vi "OpenListToINconList.vi"(11 "RVCLibrary_Bug2 in":refnum<class "RVCLibrary_Bug2.lvclass">) -> (3 "RVCLibrary_Bug2 out":refnum<class "RVCLibrary_Bug2.lvclass">)   [LabVIEW 2013, in "RVCLibrary_Bug2.lvclass"]
uses:
  RVCLibrary_Bug2.lvclass
  RVCLibrary_Bug2.lvclass/RVCLibrary_Bug2.ctl
  <vilib>/robotics/Navigation/shared/MapNode/AbstractDstarNode/NI_Robotics_AbstractDstarNode.lvclass
  <vilib>/robotics/Navigation/shared/Priority Queue/NI_Robotics_Priority Queue.lvclass
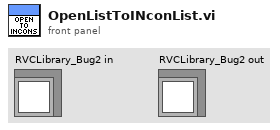
[diagram p1: front panel]
types:
  T1 = typedef "NI_Robotics_Priority Queue.lvclass/Open List Element.ctl" = cluster{"f":dbl, "g":dbl, "node Ref":refnum<data-value>}
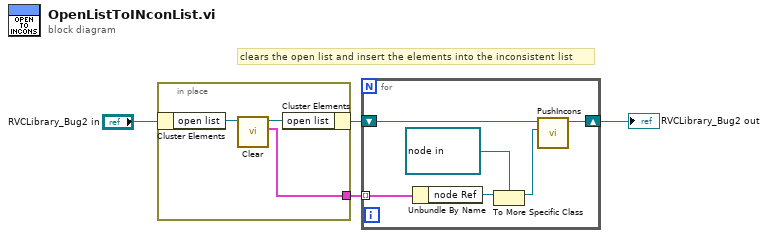
[diagram p0: block diagram]
diagram:
  # "clears the open list and insert the elements into the inconsistent list"
  n1 = in-place {
    in-place-border: [w5] -> w3
    n2 = in-place-cluster #1("RVCLibrary_Bug2 in") -> ("open list"=w7:refnum<class "NI_Robotics_Priority Queue.lvclass">)
    n3 = call <vilib>:"Clear.vi"("Priority Queue in"=w7) -> ("Open List"=w5:T1[], "Priority Queue out"=w6:refnum<class "NI_Robotics_Priority Queue.lvclass">)  [unwired: 8 in, 1 out]
    n4 = in-place-cluster #1("open list"=w6) -> (w4:refnum<class "RVCLibrary_Bug2.lvclass">)
  }
  n5 = for {
    tunnel: w3 -> [w12] mode=indexing
    shift-right: [w13] -> w2
    shift-left: w4 -> [w8]
    n6 = Unbundle By Name(w12) -> ("node Ref"=w10:refnum<data-value>)
    n7 = To More Specific Class(target class=refnum<data-value> refnum ("node ref in"), reference=w10) -> (specific class reference=w9:refnum<data-value>)  [unwired: 1 in, 1 out]
    n8 = call "PushIncons.vi"("node ref in"=w9, "RVCLibrary_Bug in"=w8) -> ("RVCLibrary_Bug out"=w13:refnum<class "RVCLibrary_Bug2.lvclass">)  [unwired: 8 in, 1 out]
  }
  "RVCLibrary_Bug2 out" <- w2
